vi "Initialize-message-queues.vi"(8 "error in (no error)":errorcluster, 11 "Object ref in":T1) -> (0 "error out":errorcluster, 3 "Object ref out":T1)   [LabVIEW 2013, in "HardwareCharacterization.lvlib" / "HC-Main.lvclass"]
uses:
  HC-Main.lvclass
  Object-reference.ctl
  Process1-actions.ctl
  Main-actions.ctl
  HC-Main.lvclass/HC-Main.ctl
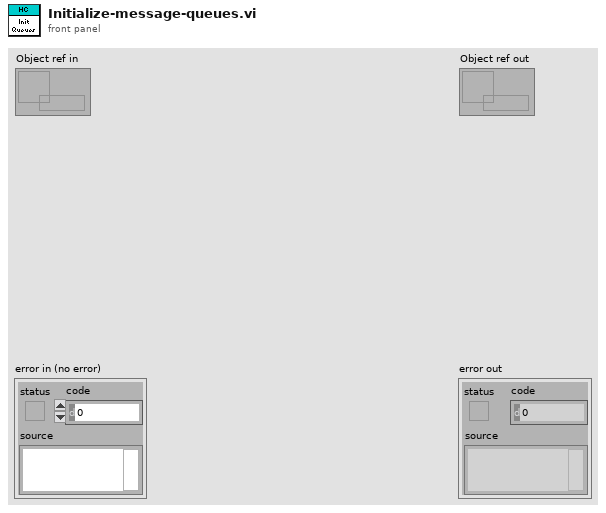
[diagram p1: front panel]
types:
  T1 = typedef "HardwareCharacterization.lvlib/HC-Main.lvclass/Object-reference.ctl" = refnum<data-value>
  T2 = typedef "HardwareCharacterization.lvlib/HC-Main.lvclass/Main-actions.ctl" = enum16{"Idle", "Initialize", "Load configuration", "Save configuration", "Load file", "Edit settings", "View scan file", "View raw path", "Edit measurement settings", "Activate", "Start", "Stop", "Refresh display", "Exit"}
  T3 = typedef "HardwareCharacterization.lvlib/HC-Main.lvclass/Process1-actions.ctl" = enum16{"Idle", "Activate", "Analyse scan file", "Convert SM1000positions", "Measure SM1000 timings", "Measure laser timings", "Stop", "Abort", "Exit"}
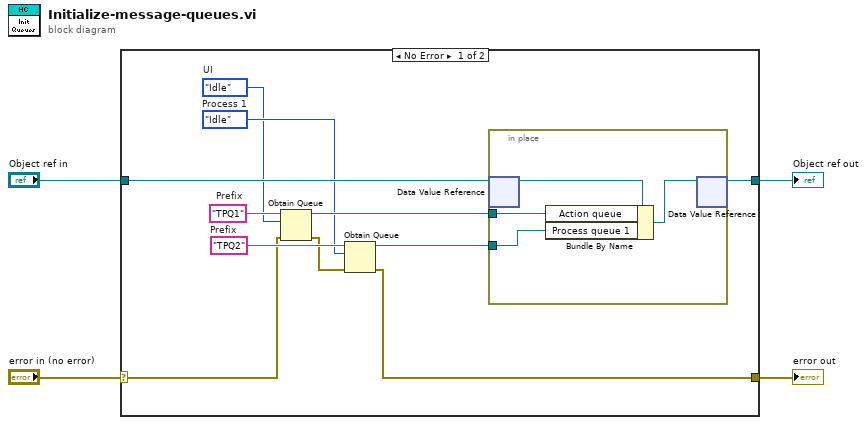
[diagram p0: block diagram]
diagram:
  n1 = case shown="No Error" "error in (no error)" {
    selector: "error in (no error)" -> [w10 w21]
    tunnel: [w5 w21] -> w3
    tunnel: [w14 w20] -> w1
    tunnel: "Object ref in" -> [w15 w20]
    frame No Error {
      w6 = Main-actions."Idle"  # UI
      w7 = Process1-actions."Idle"  # Process 1
      w12 = "TPQ2"  # Prefix
      w11 = "TPQ1"  # Prefix
      n2 = Obtain Queue(name (unnamed)=w11, element data type=w6, error in (no error)=w10) -> (queue out=w8:refnum<queue>, error out=w9:errorcluster)  [unwired: 2 in, 1 out]
      n3 = Obtain Queue(name (unnamed)=w12, element data type=w7, error in (no error)=w9) -> (queue out=w13:refnum<queue>, error out=w5:errorcluster)  [unwired: 2 in, 1 out]
      n4 = in-place {
        in-place-border: w8 -> [w17]
        in-place-border: w13 -> [w16]
        n5 = in-place-dvr #1(w15) -> (w19:refnum<class "HC-Main.lvclass">)  [unwired: 1 out]
        n6 = Bundle By Name(cluster=w19, "Action queue"=w17, "Process queue 1"=w16) -> (w18:refnum<class "HC-Main.lvclass">)
        n7 = in-place-dvr #1(w18) -> (w14:T1)  [unwired: 1 out]
      }
    }
    frame Error {
    }
  }
  "error out" <- w3
  "Object ref out" <- w1
